vi "Write Sample Push.Source Storage.vi"(6 "Publish (T)":bool=TRUE, 8 "error in (no error)":errorcluster, 10 "Source Storage (None)":T1, 11 "cRIO-CO2 in":refnum<class "cRIO-CO2.lvclass">) -> (0 "error out":errorcluster, 3 "cRIO-CO2 out":refnum<class "cRIO-CO2.lvclass">)   [LabVIEW 2015, in "cRIO-Carbondioxide.lvlib" / "cRIO-CO2.lvlib" / "cRIO-CO2.lvclass"]
uses:
  cRIO-CO2.lvclass
  Controls/Sample Transfer Container Enumerator.ctl
  cRIO-CO2.lvclass/cRIO-CO2.ctl
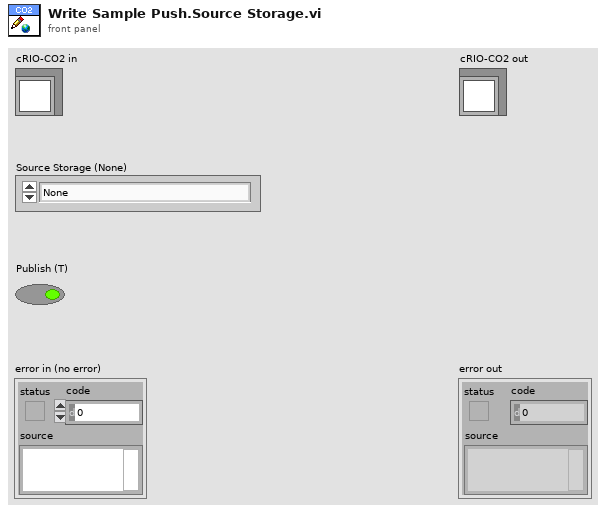
[diagram p1: front panel]
types:
  T1 = typedef "Sample Transfer Container Enumerator.ctl" = enum16{"None", "Sample 1", "Sample 2", "Sample 3", "Sample 4", "Sample 5", "Storage 01", "Storage 02", "Storage 03", "Storage 04", "Storage 05", "Storage 06", "Storage 07", "Storage 08", "Storage 09", "Storage 10", "Storage 11", "Storage 12", "Syringe", "Undefined"}
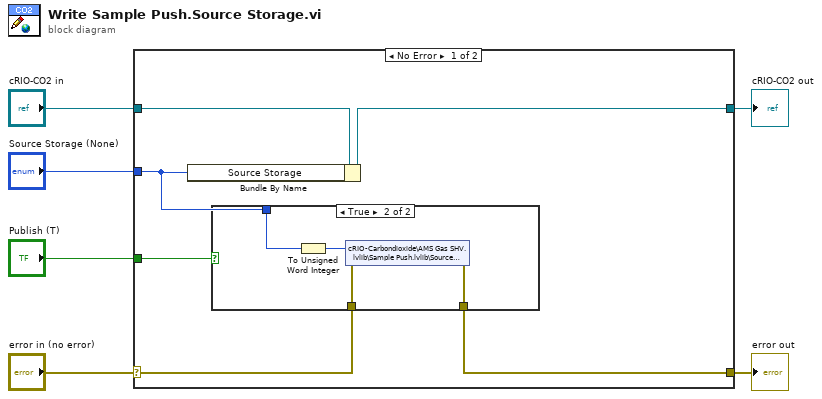
[diagram p0: block diagram]
diagram:
  n1 = case shown="No Error" "error in (no error)" {
    selector: "error in (no error)" -> [w8 w19]
    tunnel: [w7 w19] -> w5
    tunnel: [w11 w18] -> w3
    tunnel: "cRIO-CO2 in" -> [w12 w18]
    tunnel: "Publish (T)" -> [w9 _]
    tunnel: "Source Storage (None)" -> [w10 _]
    frame No Error {
      n2 = Bundle By Name(cluster=w12, "Source Storage"=w10) -> (w11:refnum<class "cRIO-CO2.lvclass">)
      n3 = case shown="True" w9 {
        tunnel: w10 -> [_ w17]
        tunnel: w8 -> [w13 w15]
        tunnel: [w13 w14] -> w7
        frame False {
        }
        frame True {
          n4 = To Unsigned Word Integer(number=w17) -> (unsigned 16bit integer=w16:u16)
          n5 = shared-variable "cRIO-Carbondioxide\\AMS Gas SHV.lvlib\\Sample Push.lvlib\\Source Storage"(w16, error in=w15) -> (error out=w14:errorcluster)
        }
      }
    }
    frame Error {
    }
  }
  "error out" <- w5
  "cRIO-CO2 out" <- w3
